vi "VisionGetNetworkTables.vi"(8 "error in (no error)":errorcluster, 11 "Vision in":refnum<class "Vision.lvclass">) -> (0 "error out":errorcluster, 2 "Cluster":T1, 3 "Vision out":refnum<class "Vision.lvclass">)   [LabVIEW 2018, in "Vision.lvlib" / "Vision.lvclass"]
doc: "tv Whether the limelight has any valid targets (0 or 1)\ntx Horizontal Offset From Crosshair To Target (-27 degrees to 27 degrees)\nty Vertical Offset From Crosshair To Target (-20.5 degrees to 20.5 degrees)\nta Target Area (0% of image to 100% of image)\nts Skew or rotation (-90 degrees to 0 degrees)\ntl The pipeline’s latency contribution (ms) Add at least 11ms for image capture latency.\ntshort Sidelength of shortest side of the fitted bounding box (pixels)\ntlong Sidelength of longest side of the fitted bounding box (pixels)\nthor Horizontal sidelength of the rough bounding box (0 - 320 pixels)\ntvert Vertical sidelength of the rough bounding box (0 - 320 pixels)\ngetpipe True active pipeline index of the camera (0 .. 9)"
uses:
  Vision.lvclass
  Controls/LimeLightData.ctl
  <vilib>/Rock Robotics/Network Tables/NT Read Numeric Array.vi
  <vilib>/Rock Robotics/Network Tables/NT Read Number.vi
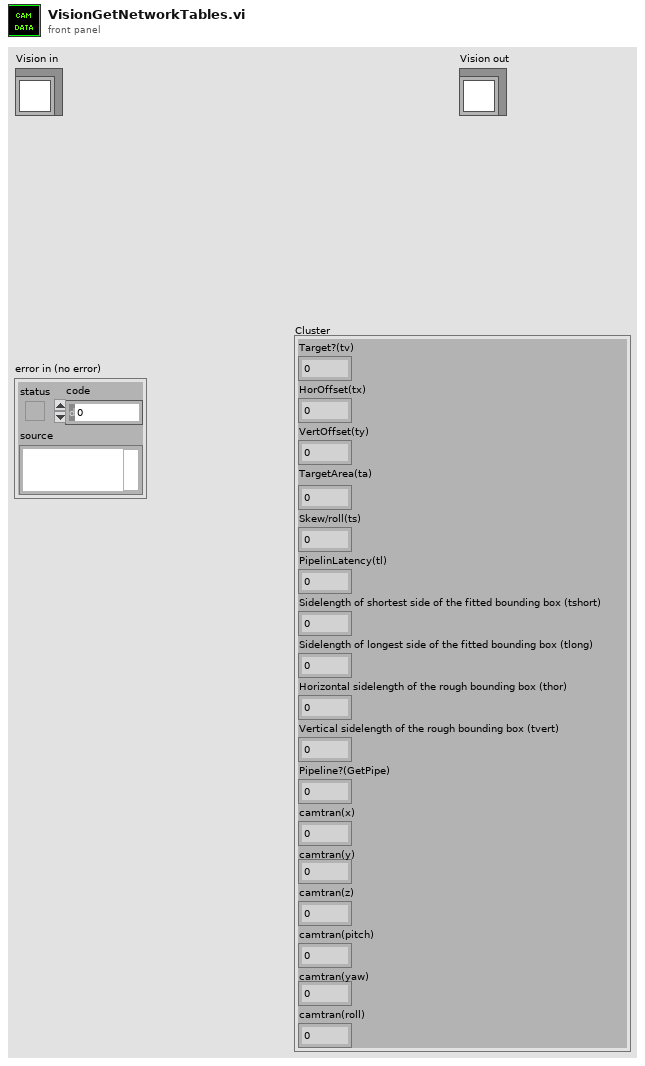
[diagram p1: front panel]
types:
  T1 = typedef "Vision.lvlib/Vision.lvclass/LimeLightData.ctl" = cluster{"Target?(tv)":dbl, "HorOffset(tx)":dbl, "VertOffset(ty)":dbl, "TargetArea(ta)":dbl, "Skew/roll(ts)":dbl, "PipelinLatency(tl)":dbl, "Sidelength of shortest side of the fitted bounding box (tshort) ":dbl, "Sidelength of longest side of the fitted bounding box (tlong)":dbl, "Horizontal sidelength of the rough bounding box (thor)":dbl, "Vertical sidelength of the rough bounding box (tvert)":dbl, "Pipeline?(GetPipe)":dbl, "camtran(x)":dbl, "camtran(y)":dbl, "camtran(z)":dbl, "camtran(pitch)":dbl, "camtran(yaw)":dbl, "camtran(roll)":dbl}
  T2 = cluster{"[0]":dbl, "[1]":dbl, "[2]":dbl, "[3]":dbl, "[4]":dbl, "[5]":dbl, "[6]":dbl, "[7]":dbl, "[8]":dbl, "[9]":dbl, "[10]":dbl, "[11]":dbl, "[12]":dbl, "[13]":dbl, "[14]":dbl, "[15]":dbl, "[16]":dbl}
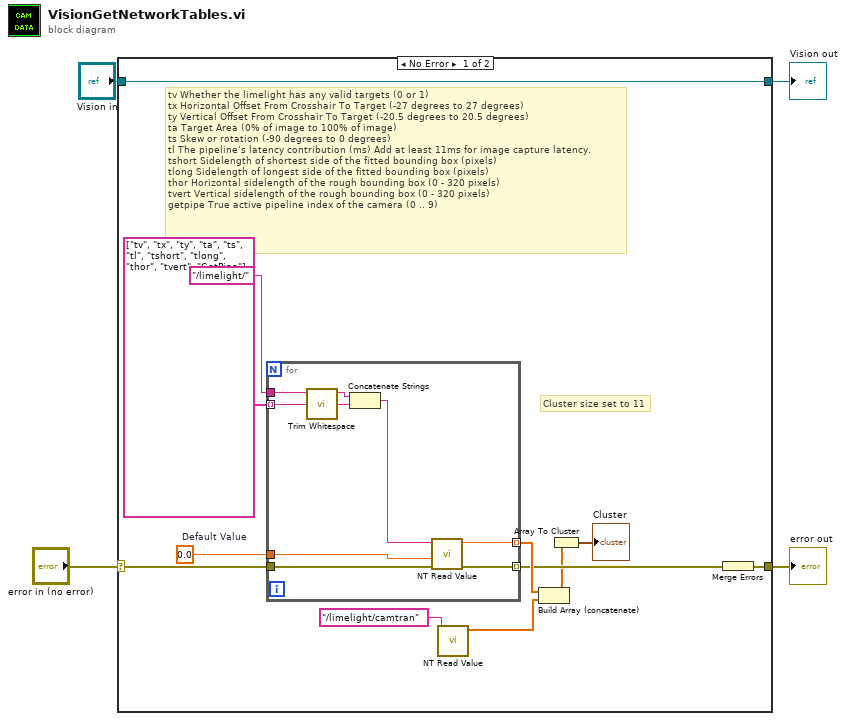
[diagram p0: block diagram]
diagram:
  n1 = case shown="No Error" "error in (no error)" {
    selector: "error in (no error)" -> [w10 w26]
    tunnel: [w8 w26] -> w3
    tunnel: [w16 w25] -> w1
    tunnel: "Vision in" -> [w16 w25]
    frame No Error {
      w15 = 0.0  # Default Value
      # "Cluster size set to 11"
      # "tv\tWhether the limelight has any valid targets (0 or 1)\ntx\tHorizontal Offset From Crosshair To Target (-27 degrees to 27 degrees)\nty\tVertical Offset From Crosshair To Target (-20.5 degrees to 20.5 degrees)\nta\tTarget Area (0% of image to 100% of image)\nts\tSkew or rotation (-90 degrees to 0 degrees)\ntl\tThe pipeline’s latency contribution (ms) Add at least 11ms for image capture latency.\ntshort\tSidelength of shortest side of the fitted bounding box (pixels)\ntlong\tSidelength of longest side of the fitted bounding box (pixels)\nthor\tHorizontal sidelength of the rough bounding box (0 - 320 pixels)\ntvert\tVertical sidelength of the rough bounding box (0 - 320 pixels)\ngetpipe\tTrue active pipeline index of the camera (0 .. 9)"
      n2 = for {
        tunnel: w15 -> [w24]
        tunnel: "/limelight/" ("Name") -> [w23]
        tunnel: [w21] -> w13 mode=indexing
        tunnel: string[] ["tv", "tx", "ty", "ta", "ts", "tl", "tshort", "tlong", "thor", "tvert", "GetPipe"] -> [w20] mode=indexing
        tunnel: w10 -> [w19]
        tunnel: [w18] -> w9 mode=indexing
        n3 = call <vilib>:"Trim Whitespace.vi"("string"=w20) -> ("trimmed string"=w17:string)  [unwired: 1 in]
        n4 = Concatenate Strings(w23, w17) -> (w22:string)
        n5 = call-poly <vilib>:"NT Read Value.vi"("error in"=w19, "Default Value"=w24, "Name"=w22) -> ("error out"=w18:errorcluster, "Numeric"=w21:dbl)  [unwired: 7 in]
      }
      n6 = call-poly <vilib>:"NT Read Value.vi"("Name"="/limelight/camtran") -> ("Numeric Array"=w6:dbl[])  [unwired: 9 in, 1 out]
      n7 = Build Array (concatenate)(w13, w6) -> (w7:dbl[])
      n8 = Array To Cluster(array=w7) -> (cluster=→"Cluster":T2)
      n9 = Merge Errors(w9) -> (w8:errorcluster)
    }
    frame Error {
    }
  }
  "error out" <- w3
  "Vision out" <- w1
